vi "Cache_Hierarchy Global_Load All.vi"(8 "error in (no error)":errorcluster) -> (0 "error out":errorcluster, 3 "Hierarchy Map":map{string, string[]}(c390))   [LabVIEW 2020, in "ClassLoader.lvlib"]
doc: "Return paths to the ini cache files for all loaded PPLs."
uses:
  ClassLoader.lvlib
  Cache_Hierarchy Global.vi
  <vilib>/Utility/config.llb/NI_LVConfig.lvlib
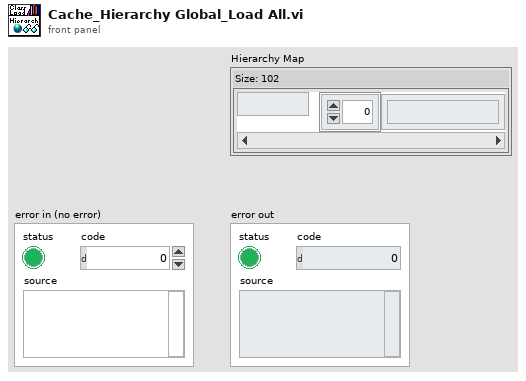
[diagram p1: front panel]
types:
  T1 = typedef "NI_LVConfig.lvlib/Config Data RefNum.ctl" = refnum<k1>
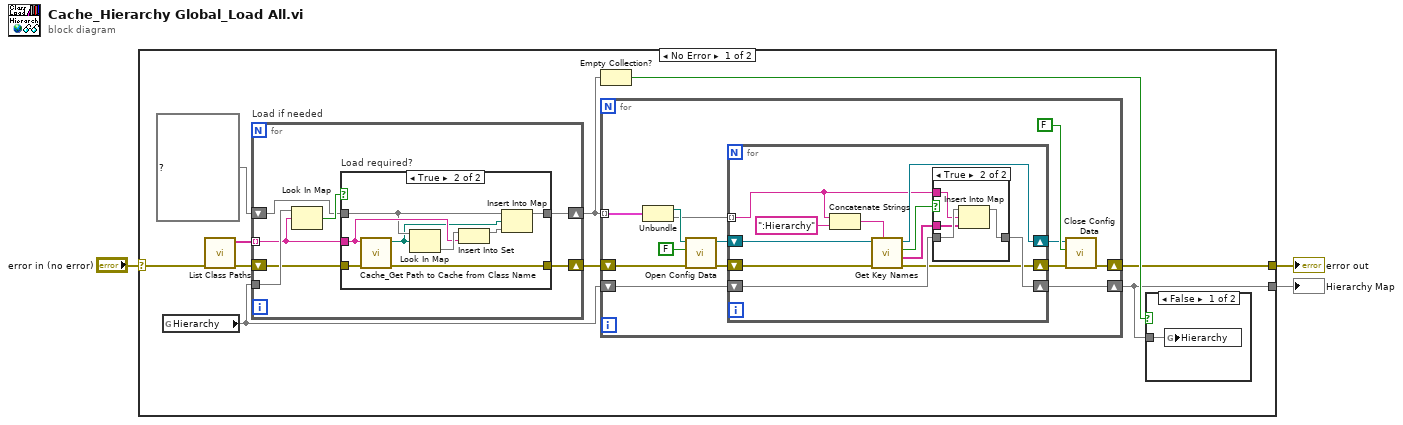
[diagram p0: block diagram]
diagram:
  n1 = case shown="No Error" "error in (no error)" {
    selector: "error in (no error)" -> [w13 w61]
    tunnel: [w5 w61] -> w2
    tunnel: [w4 _] -> w1
    frame No Error {
      n2 = global read "Cache_Hierarchy Global.vi" "Hierarchy"() -> (w8:map{string, string[]})
      n3 = call "List Class Paths.vi"("error in (no error)"=w13) -> ("error out"=w9:errorcluster, "Class Names"=w12:string[])  [unwired: 8 in, 1 out]
      n4 = for "Load if needed" {
        tunnel: w12 -> [w48] mode=indexing
        tunnel: w8 -> [w49]
        shift-right: [w46] -> w7
        shift-left: map{path, set{string}} {} ("map") -> [w47]
        shift-right: [w45] -> w10
        shift-left: w9 -> [w44]
        n5 = Look In Map(map=w49, key=w48) -> (key not found?=w50:bool)  [unwired: 1 in, 1 out]
        n6 = case "Load required?" shown="True" w50 {
          tunnel: w48 -> [_ w59]
          tunnel: w47 -> [w52 w58]
          tunnel: [w52 w57] -> w46
          tunnel: [w51 w53] -> w45
          tunnel: w44 -> [w51 w54]
          frame False {
          }
          frame True {
            n7 = call "Cache_Get Path to Cache from Class Name.vi"("error in (no error)"=w54, "Class Name"=w59) -> ("error out"=w53:errorcluster, "Cache Path"=w56:path)  [unwired: 7 in, 1 out]
            n8 = Look In Map(map=w58, key=w56) -> (value=w60:set{string})  [unwired: 1 in, 1 out]
            n9 = Insert Into Set(10:w59, 11:w60) -> (3:w55:set{string})  [unwired: 1 out]
            n10 = Insert Into Map(map in=w58, key=w56, value=w55) -> (map out=w57:map{path, set{string}})  [unwired: 2 out]
          }
        }
      }
      n11 = Empty Collection?(1:w7) -> (0:w6:bool)
      n12 = for {
        tunnel: w7 -> [w27] mode=indexing
        shift-right: [w17] -> w5
        shift-left: w10 -> [w24]
        shift-right: [w15] -> w4
        shift-left: w8 -> [w16]
        n13 = Unbundle(w27) -> ("Cache Path"=w25:path, "set"=w21:set{string})
        n14 = call <vilib>:"Open Config Data.vi"("error in (no error)"=w24, "create file if necessary (T)"=FALSE, "configuration file path"=w25) -> ("error out"=w19:errorcluster, "refnum"=w22:T1)  [unwired: 6 in, 1 out]
        n15 = for {
          shift-right: [w35] -> w20
          shift-left: w22 -> [w37]
          tunnel: w21 -> [w28] mode=indexing
          shift-right: [w29] -> w18
          shift-left: w19 -> [w34]
          shift-right: [w32] -> w15
          shift-left: w16 -> [w31]
          n16 = Concatenate Strings(w28, ":Hierarchy" ("string")) -> (w36:string)
          n17 = call <vilib>:"Get Key Names.vi"("section"=w36, "error in (no error)"=w34, "refnum"=w37) -> ("error out"=w29:errorcluster, "key names"=w30:string[], "section exists?"=w33:bool, "refnum out"=w35:T1)  [unwired: 5 in]
          n18 = case shown="True" w33 {
            tunnel: [w39 w41] -> w32
            tunnel: w31 -> [w39 w43]
            tunnel: w30 -> [_ w42]
            tunnel: w28 -> [_ w40]
            frame False {
            }
            frame True {
              n19 = Insert Into Map(map in=w43, key=w40, value=w42) -> (map out=w41:map{string, string[]})  [unwired: 2 out]
            }
          }
        }
        n20 = call <vilib>:"Close Config Data.vi"("error in (no error)"=w18, "write file if changed (T)"=FALSE, "refnum"=w20) -> ("error out"=w17:errorcluster)  [unwired: 7 in, 1 out]
      }
      n21 = case shown="False" w6 {
        tunnel: w4 -> [w14 _]
        frame False {
          n22 = global write "Cache_Hierarchy Global.vi" "Hierarchy"(w14) -> ()
        }
        frame True {
        }
      }
    }
    frame Error {
    }
  }
  "error out" <- w2
  "Hierarchy Map" <- w1
